vi "Grain Boundary Genie - Copy.vi"() -> ()   [LabVIEW 2010]
uses:
  <vilib>/Analysis/NI_AALBase.lvlib
  <vilib>/Analysis/baseanly.llb/Real Dot Product.vi
  <vilib>/Analysis/NI_AALPro.lvlib
  <vilib>/Analysis/_algsub.llb/Real Vector Norm.vi
  <vilib>/picture/3D Picture Control/NI_3D Picture Control.lvlib
  <vilib>/Analysis/baseanly.llb/Real A x B.vi
  <vilib>/Analysis/baseanly.llb/Vector x A.vi
  <vilib>/Utility/file.llb/Write To Spreadsheet File (string).vi
panel:
  in  "Grain 2 Max Length (A)":dbl=10.0
  in  "Grain 1 Max Length (A)":dbl=10.0
  in  "Max Grain Width":dbl=100.0
  in  "Grain 1 Start":dbl
  in  "Conventional Unit Cell":T1={"Structure Name"="CdTe", "Lattice vector a"=[6.615785553057252, 0.0, 0.0], "Lattice vector b"=[0.0, 6.615785553057252, 0.0], "Lattice vector c"=[0.0, 0.0, 6.615785553057252], "Atoms Array"=[{"Atom Name"="Cd", "Positions (Direct)"=[[0.0, 0.0, 0.0], [0.0, 0.5, 0.5], [0.5, 0.0, 0.5], [0.5, 0.5, 0.0]], "Positions (Cartesian)"=[[0.0, 0.0, 0.0], [0.0, 3.307892776528626, 3.307892776528626], [3.307892776528626, 0.0, 3.307892776528626], [3.307892776528626, 3.307892776528626, 0.0]]}, {"Atom Name"="Te", "Positions (Direct)"=[[0.25, 0.25, 0.25], [0.75, 0.75, 0.25], [0.75, 0.25, 0.75], [0.25, 0.75, 0.75]], "Positions (Cartesian)"=[[1.653946388264313, 1.653946388264313, 1.653946388264313], [4.96183916479294, 4.96183916479294, 1.653946388264313], [4.96183916479294, 1.653946388264313, 4.96183916479294], [1.653946388264313, 4.96183916479294, 4.96183916479294]]}], "# of atoms"=8}
  in  "Overlap Region (A)":dbl(slide) scale=-2.0..1.0
  in  "Tab Control":T2(tab)
  in  "Remove Close Atoms":bool
  out "Subset for Y?":bool
  out "Repeating Y Length Scale":dbl=99.01964045547014
  in  "Crop to Smallest Repeating":bool
  in  "Slab Y":dbl=6.0
  in  "Slab X":dbl=6.0
  out "Subset for X?":bool
  in  "Tolerance (A)":dbl=1.0
  in  "Presorted?":bool
  out "Repeating X Length Scale":dbl=99.01964045547014
  in  "Minimally Allowable Distance (A)":dbl=1.5
  out "# of Atoms Removed":i32
  in  "Make GB":bool
  in  "Options":cluster{"Border?":bool, "Bonds?":bool}={"Border?"=TRUE, "Bonds?"=FALSE}
  in  "Scale":dbl(slide)=0.06161137440758294 scale=0.0..0.2
  in  "Mutual Viewing Angle":dbl[](array[numeric])=[1.0, 0.0, 0.0]
  out "# of Atoms":i32
  out "Atoms / A³":dbl
  out "% of Bulk atomic density":dbl
  in  "Structure Name":string
  in  "Save to POSCAR":bool
  out "Grain Boundary Object":refnum<vi>
  out "Grain 2 Object":refnum<vi>
  out "Grain 1 Object":refnum<vi>
  in  "Add Tilt Angle":dbl(slide) scale=0.0..90.0
  out "Grain Boundary":T1={"Structure Name"="Relax2 Subcrystal Expanded to Box+Relax2 Subcrystal Expanded to Box", "Lattice vector a"=[10.1, 0.0, 0.0], "Lattice vector b"=[0.0, 100.1, 0.0], "Lattice vector c"=[0.0, 0.0, 24.72380952380952], "Atoms Array"=[{"Atom Name"="Cd", "Positions (Direct)"=array496x3[1488 elements], "Positions (Cartesian)"=array496x3[1488 elements]}, {"Atom Name"="Te", "Positions (Direct)"=array480x3[1440 elements], "Positions (Cartesian)"=array480x3[1440 elements]}], "# of atoms"=976} {"Atoms Array"."Positions (Cartesian)" format="%#_4f"; "Atoms Array"."Positions (Direct)" format="%#_4f"}
  out "Grain 2":T1={"Structure Name"="Relax2 Subcrystal Expanded to Box", "Lattice vector a"=[10.1, 0.0, 0.0], "Lattice vector b"=[0.0, 100.1, 0.0], "Lattice vector c"=[0.0, 0.0, 10.1], "Atoms Array"=[{"Atom Name"="Cd", "Positions (Direct)"=array248x3[744 elements], "Positions (Cartesian)"=array248x3[744 elements]}, {"Atom Name"="Te", "Positions (Direct)"=array240x3[720 elements], "Positions (Cartesian)"=array240x3[720 elements]}], "# of atoms"=488} {"Atoms Array"."Positions (Cartesian)" format="%#_4f"; "Atoms Array"."Positions (Direct)" format="%#_4f"}
  out "Grain 1":T1={"Structure Name"="Relax2 Subcrystal Expanded to Box", "Lattice vector a"=[10.1, 0.0, 0.0], "Lattice vector b"=[0.0, 100.1, 0.0], "Lattice vector c"=[0.0, 0.0, 10.1], "Atoms Array"=[{"Atom Name"="Cd", "Positions (Direct)"=array248x3[744 elements], "Positions (Cartesian)"=array248x3[744 elements]}, {"Atom Name"="Te", "Positions (Direct)"=array240x3[720 elements], "Positions (Cartesian)"=array240x3[720 elements]}], "# of atoms"=488} {"Atoms Array"."Positions (Cartesian)" format="%#_4f"; "Atoms Array"."Positions (Direct)" format="%#_4f"}
  in  "Primitive Lattice Vectors":T1={"Structure Name"="Relax2 Subcrystal", "Lattice vector a"=[0.0, 3.3046962263585, 3.3046962263585], "Lattice vector b"=[3.3046962263585, 0.0, 3.3046962263585], "Lattice vector c"=[3.3046962263585, 3.3046962263585, 0.0], "Atoms Array"=[{"Atom Name"="Cd", "Positions (Direct)"=[[0.0, 0.0, 0.0]], "Positions (Cartesian)"=[[0.0, 0.0, 0.0]]}, {"Atom Name"="Te", "Positions (Direct)"=[[0.25, 0.25, 0.25]], "Positions (Cartesian)"=[[1.65234811317925, 1.65234811317925, 1.65234811317925]]}], "# of atoms"=2} {"Atoms Array"."Positions (Cartesian)" format="%#_4f"; "Atoms Array"."Positions (Direct)" format="%#_4f"}
  in  "Grain 2 Min Length (A)":dbl=10.0
  in  "Grain 1 Min Length (A)":dbl=10.0
  out "Grain Boundary Render":refnum<vi>(3d-picture)
  in  "Max Grain Height":dbl=100.0
  in  "Translation Vector":dbl[](array[slide])=[0.0, 0.0, 4.523809523809524] scale=0.0..2.0
  in  "Twist Angle":dbl(slide)=60.0 scale=0.0..60.0
  in  "Grain 2 Orientation":dbl[](array[numeric])=[1.0, 0.0, 0.0]
  in  "Grain 1 Orientation":dbl[](array[numeric])=[1.0, 0.0, 0.0]
  out "Grain 2 Render":refnum<vi>(3d-picture)
  out "Grain 1 Render":refnum<vi>(3d-picture)
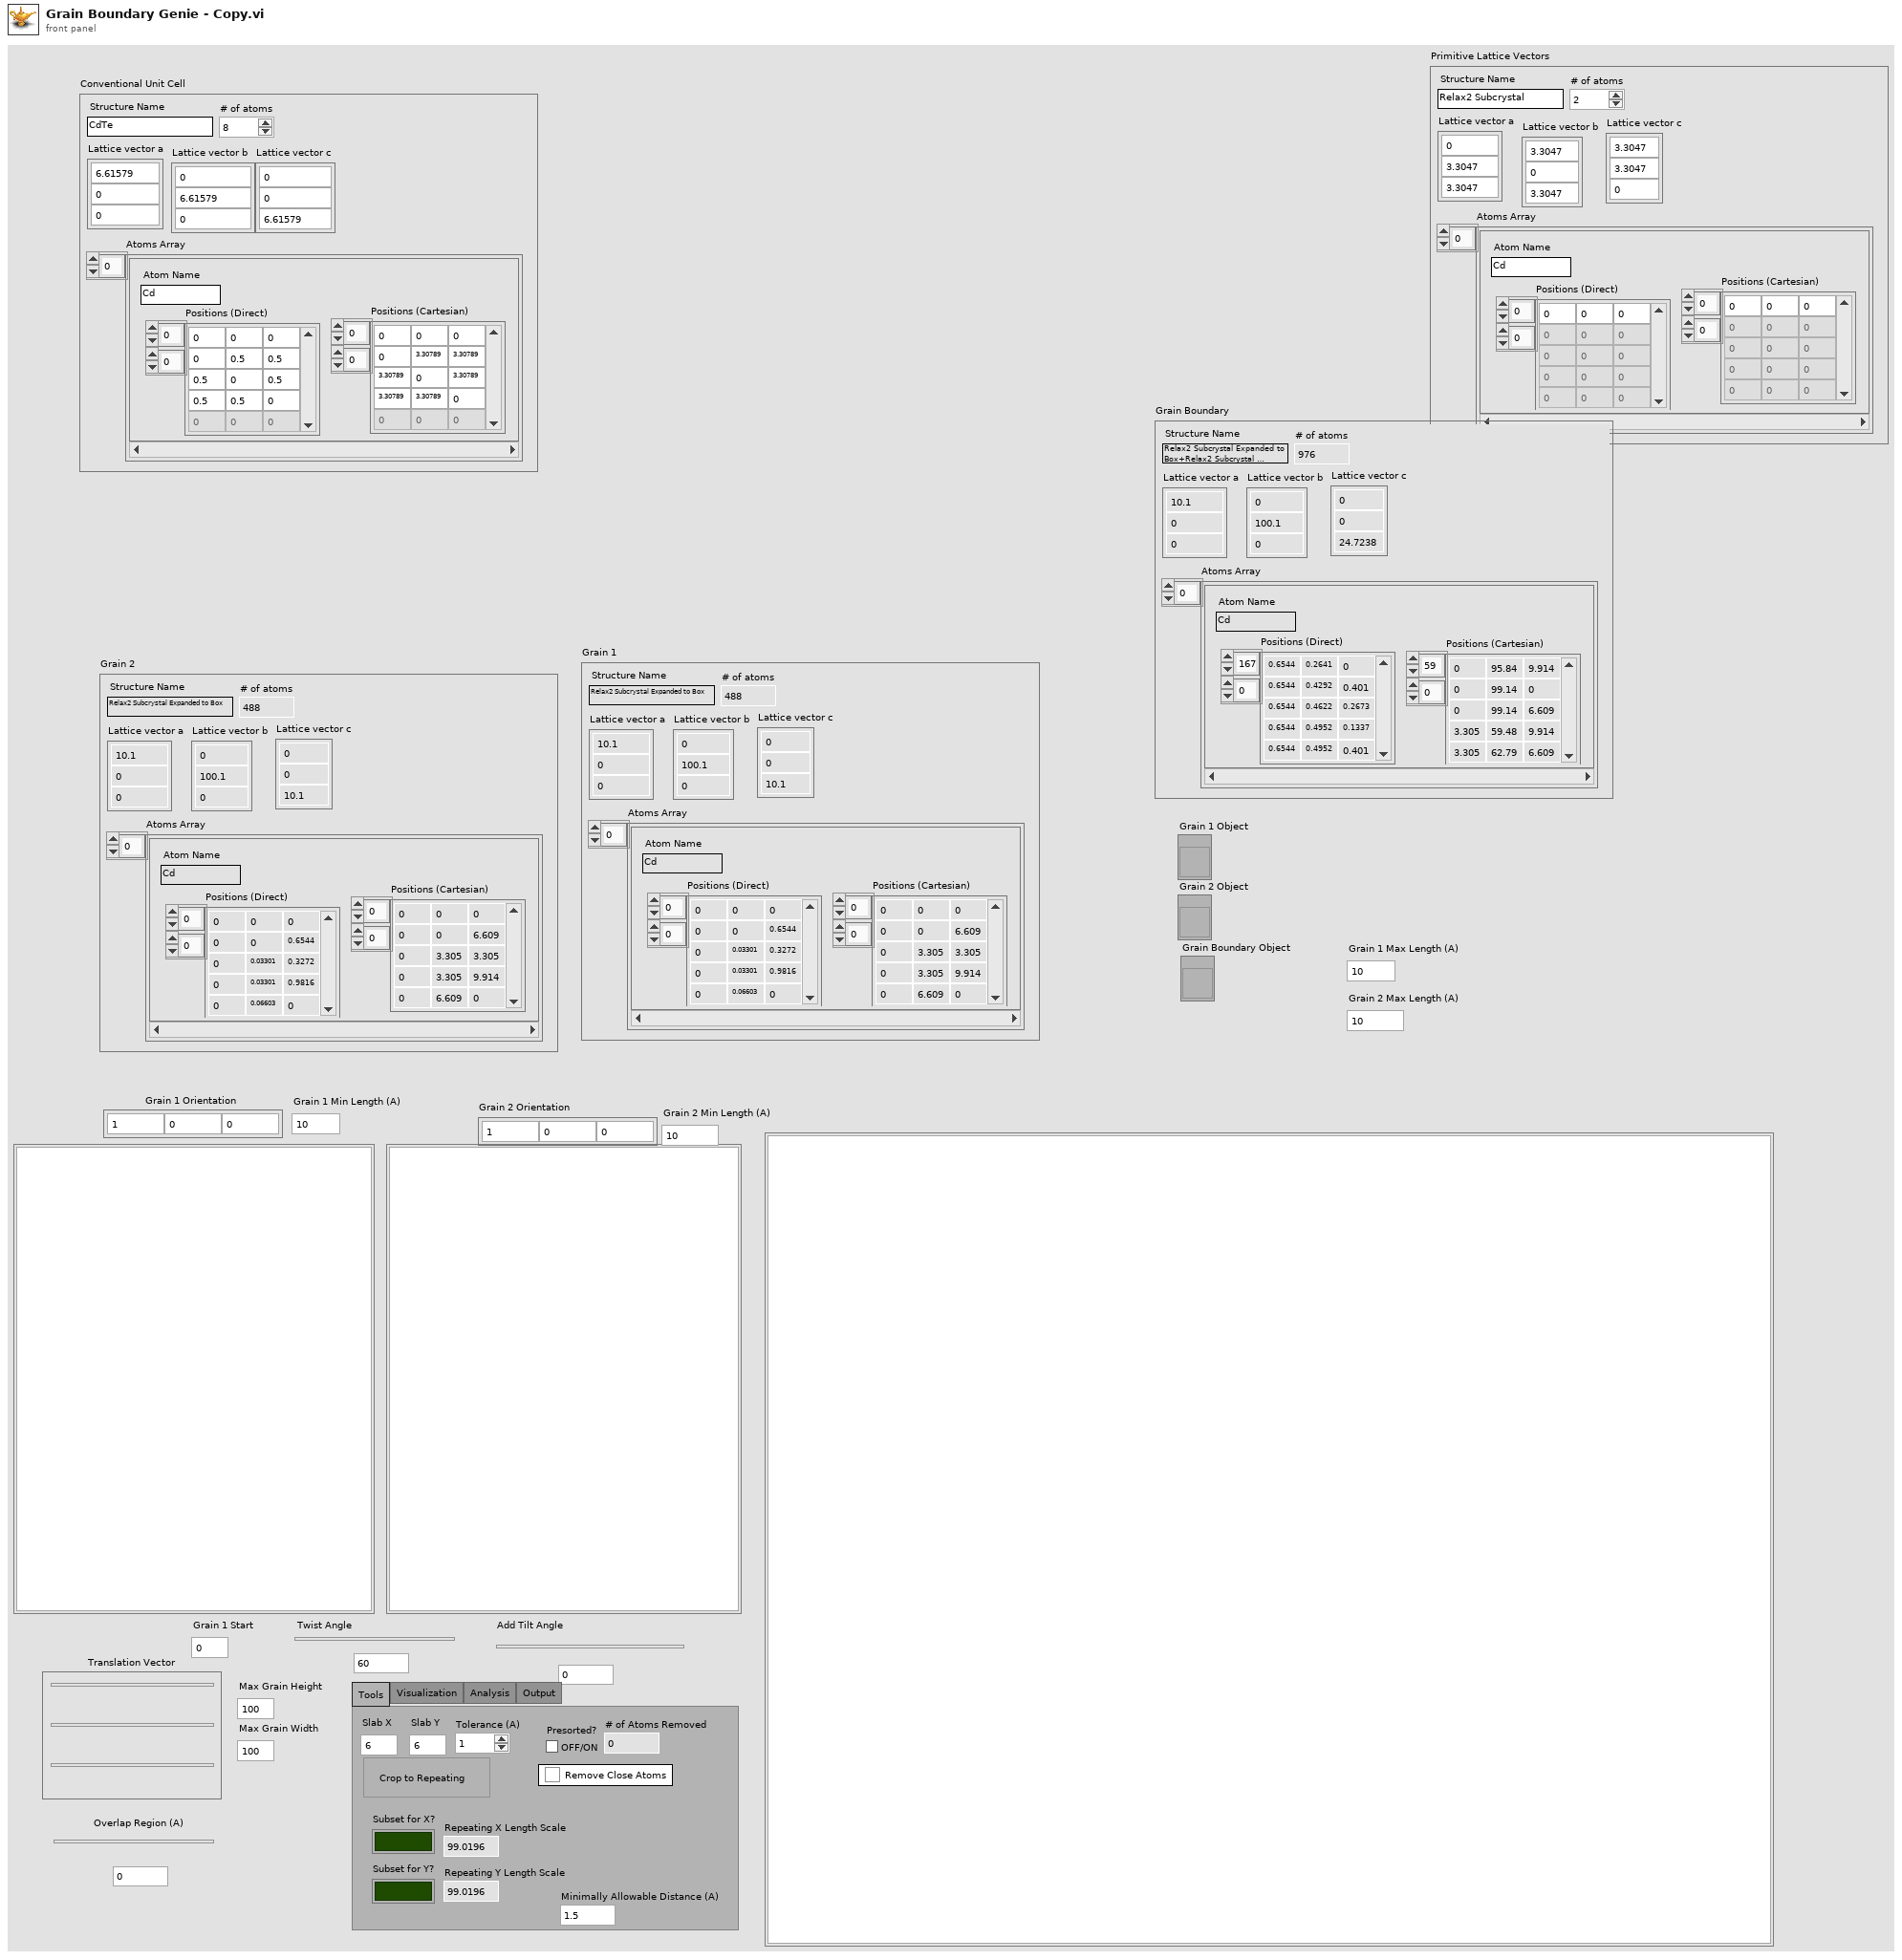
[diagram p1: front panel]
types:
  T1 = cluster{"Structure Name":string, "Lattice vector a":dbl[], "Lattice vector b":dbl[], "Lattice vector c":dbl[], "Atoms Array":cluster{"Atom Name":string, "Positions (Direct)":dbl[][], "Positions (Cartesian)":dbl[][]}[], "# of atoms":i32}
  T2 = enum32{"Tools", "Visualization", "Analysis", "Output"}
  T3 = typedef "NI_Matrix.lvlib/RealMatrix.ctl" = dbl[][]
  T4 = cluster{"Z Min":dbl, "Max Grain Width":dbl, "Z Min":dbl, "Max Grain Height":dbl, "Grain 1 Start":dbl, "Grain 1 Min Length (A)":dbl}
  T5 = cluster{"Grain 1 Start":dbl, "Max Grain Width":dbl, "Grain 1 Start":dbl, "Max Grain Height":dbl, dbl, "Grain 2 Min Length (A)":dbl}
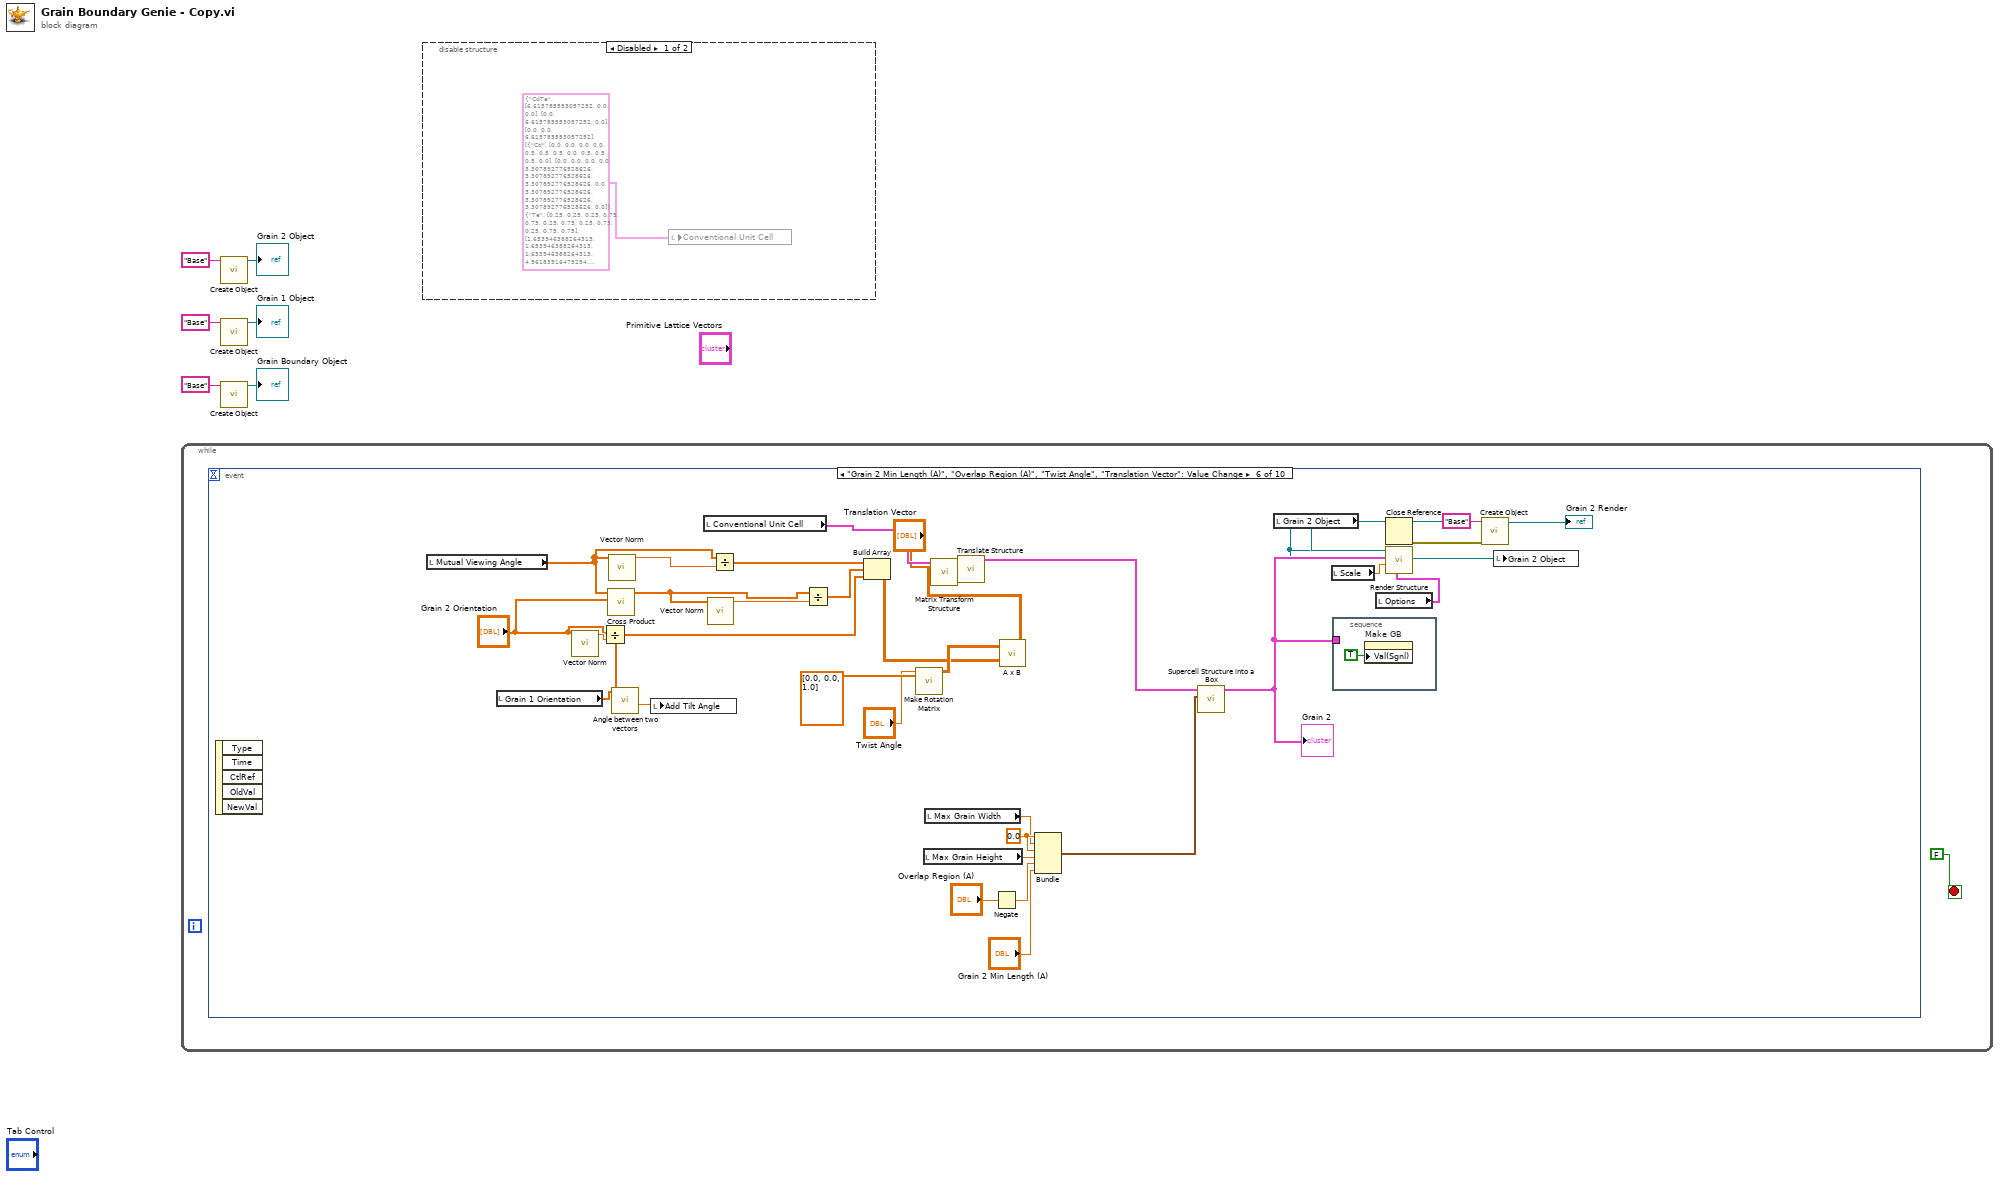
[diagram p0: block diagram]
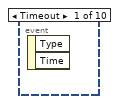
[diagram p3: hidden frame]
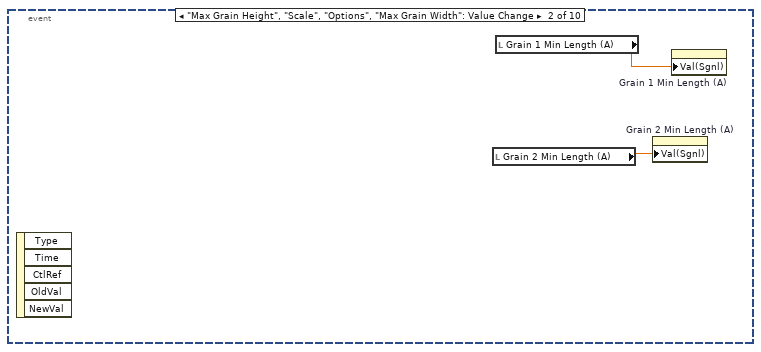
[diagram p4: hidden frame]
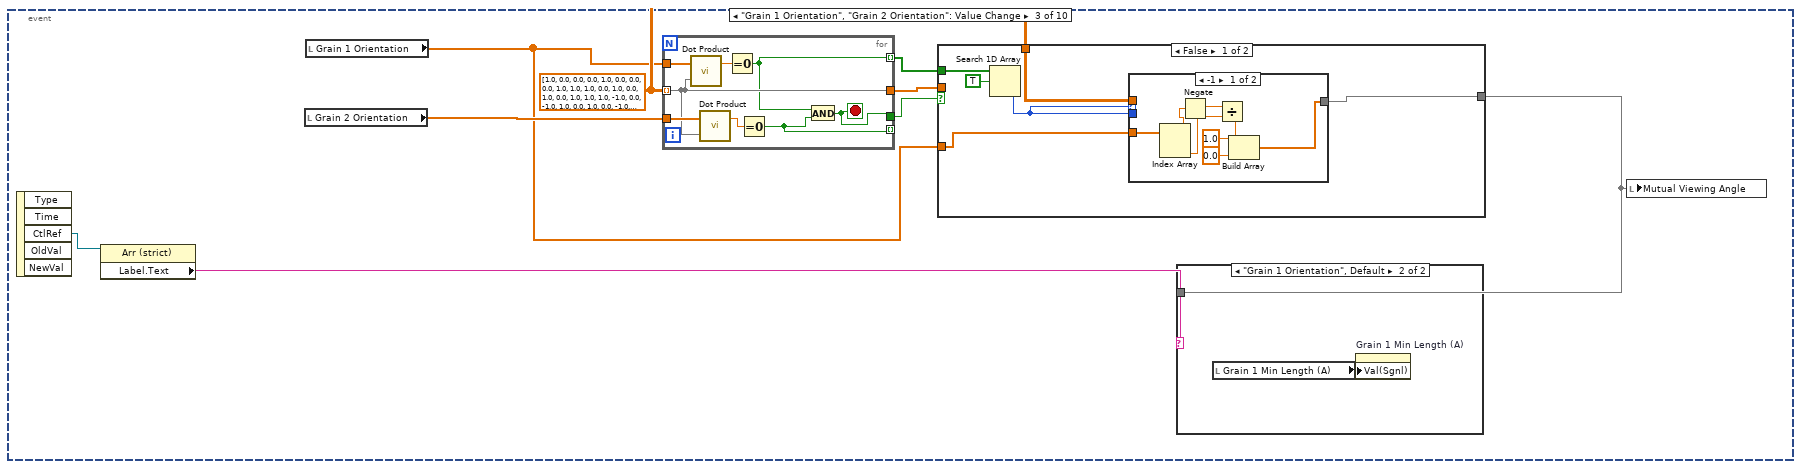
[diagram p5: hidden frame]
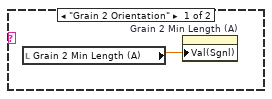
[diagram p6: hidden frame]
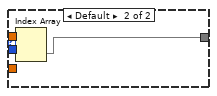
[diagram p7: hidden frame]
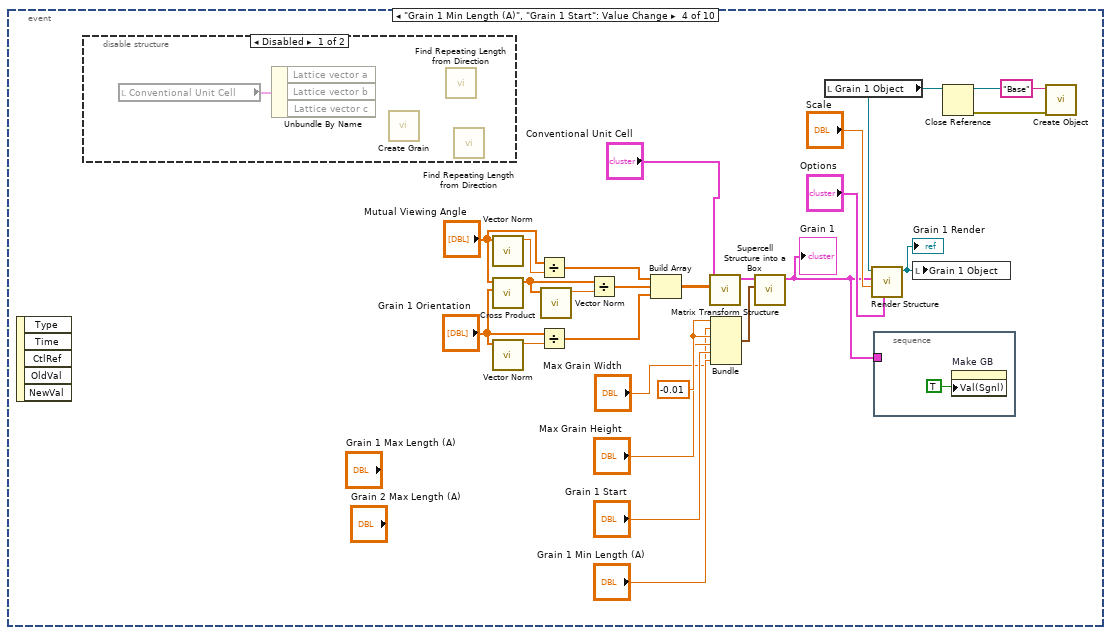
[diagram p9: hidden frame]
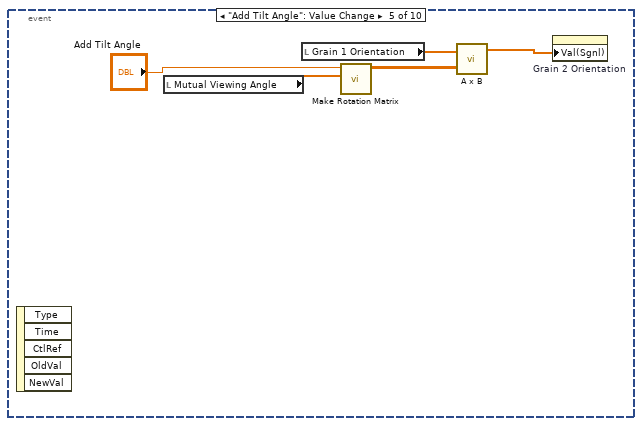
[diagram p11: hidden frame]
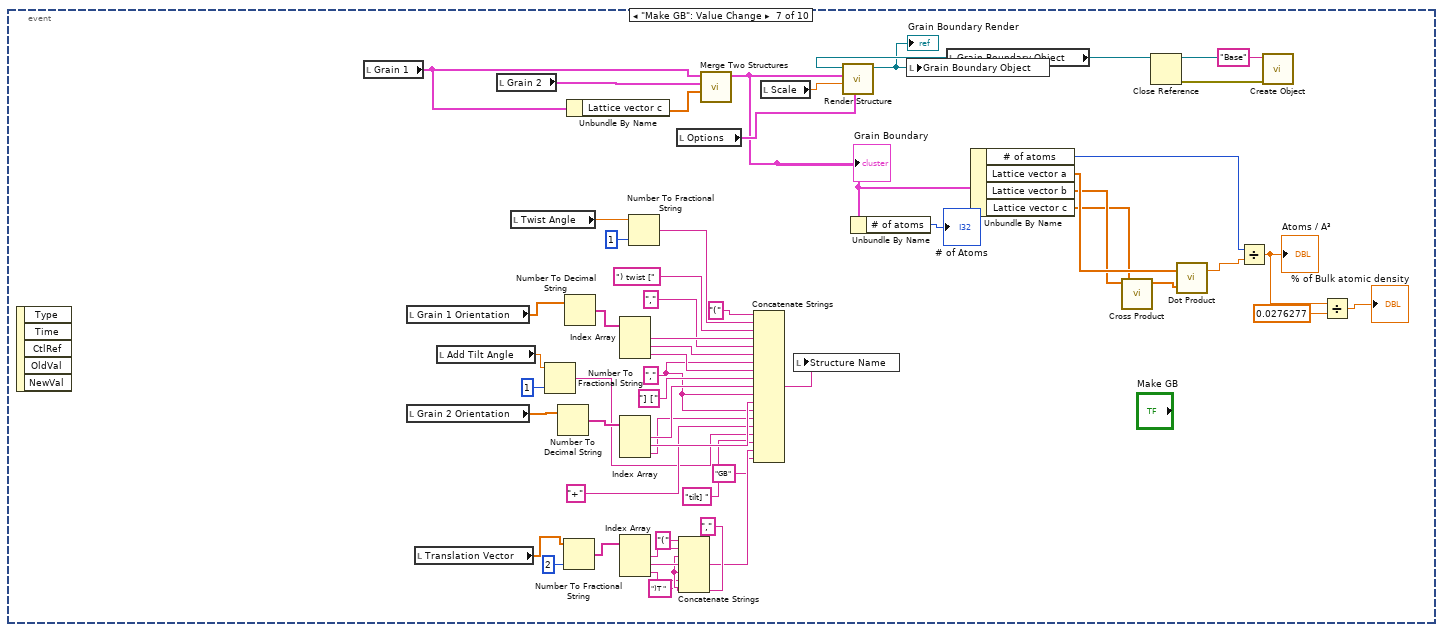
[diagram p12: hidden frame]
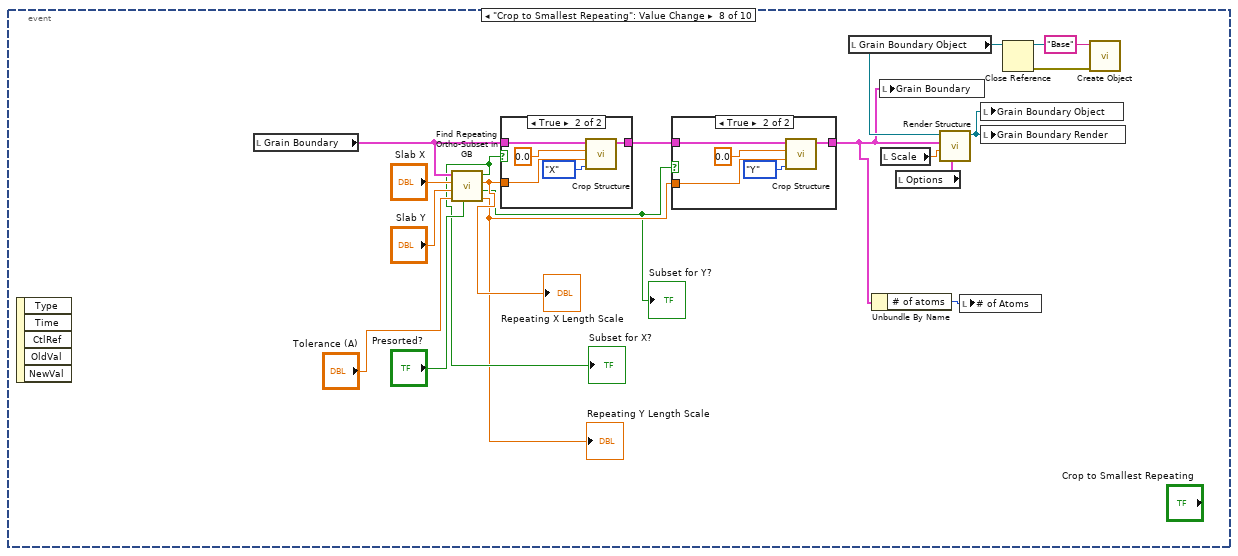
[diagram p13: hidden frame]
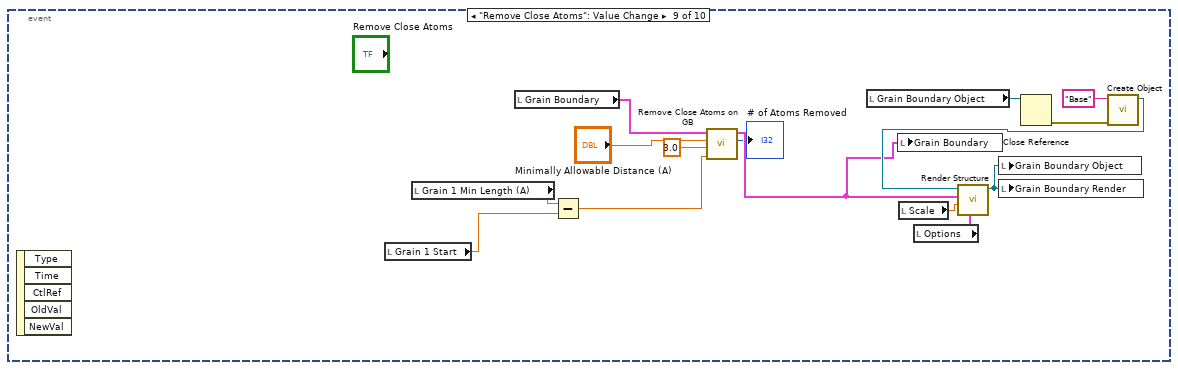
[diagram p16: hidden frame]
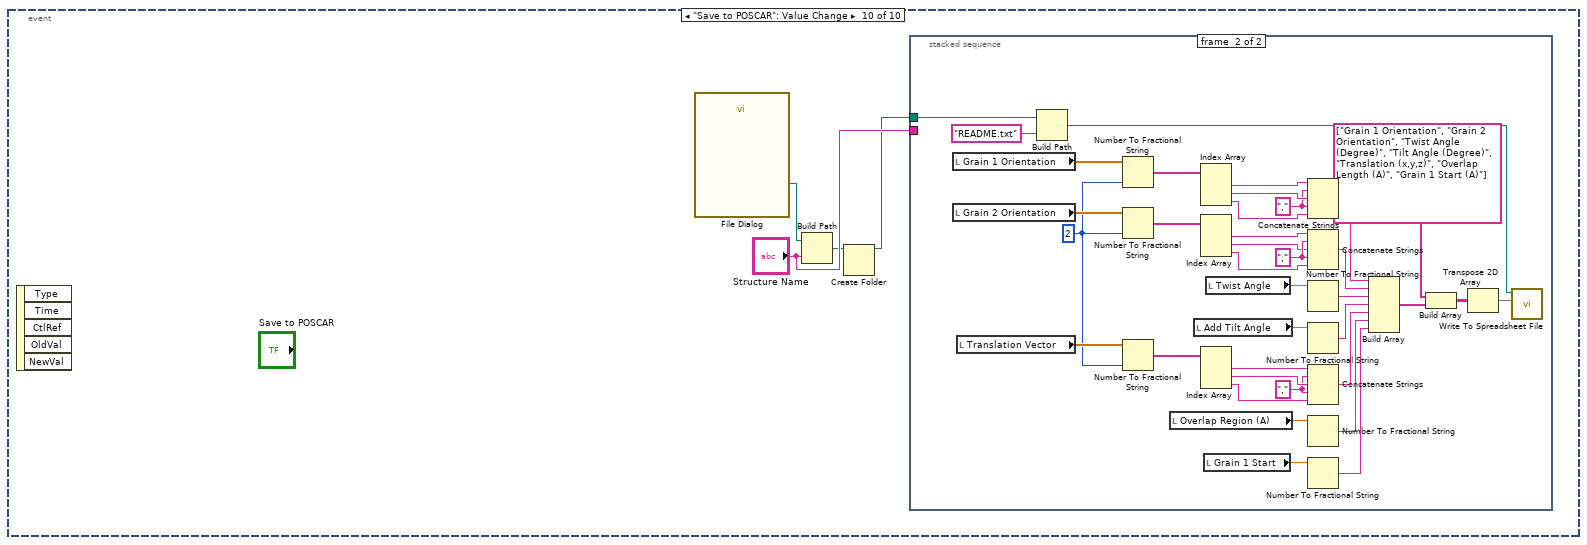
[diagram p17: hidden frame]
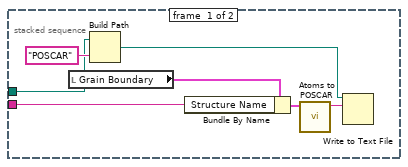
[diagram p18: hidden frame]
diagram:
  n1 = while {
    stop <- FALSE stop-if-true
    n2 = event shown="[5] \"Grain 2 Min Length (A)\", \"Overlap Region (A)\", \"Twist Angle\", \"Translation Vector\": Value Change" {
      selector: _ -> [_ _ _ _ _ _ _ _ _ _]
      dyn-events: _ -> [_ _ _ _ _ _ _ _ _ _]
      timeout: _ -> [_ _ _ _ _ _ _ _ _ _]
      event Timeout {
        n3 = event-data() -> ()  [unwired: 1 in, 2 out]
      }
      event "Max Grain Height", "Scale", "Options", "Max Grain Width": Value Change {
        n4 = event-data() -> ()  [unwired: 1 in, 5 out]
        n5 = local read "Grain 2 Min Length (A)"() -> (w8:dbl)
        n6 = local read "Grain 1 Min Length (A)"() -> (w9:dbl)
        n7 = property on="Grain 2 Min Length (A)" class="DigNum (strict)"("Val(Sgnl)"=w8) -> ()  [unwired: 2 in, 2 out]
        n8 = property on="Grain 1 Min Length (A)" class="DigNum (strict)"("Val(Sgnl)"=w9) -> ()  [unwired: 2 in, 2 out]
      }
      event "Grain 1 Orientation", "Grain 2 Orientation": Value Change {
        w14 = dbl[][] [[1.0, 0.0, 0.0], [0.0, 1.0, 0.0], [0.0, 0.0, 1.0], [1.0, 1.0, 0.0], [1.0, 0.0, 1.0], [0.0, 1.0, 1.0], [1.0, -1.0, 0.0], [-1.0, 1.0, 0.0], [1.0, 0.0, -1.0], [-1.0, 0.0, 1.0], [0.0, -1.0, 1.0], [0.0, 1.0, -1.0], [2.0, 1.0, 0.0], [2.0, 1.0, 1.0]] ("Grain 1 Orientation 2")
        n9 = event-data() -> ("CtlRef"=w13:refnum<vi>)  [unwired: 1 in, 4 out]
        n10 = property class="Arr (strict)"(reference=w13) -> ("Label.Text"=w12:string)  [unwired: 1 in, 2 out]
        n11 = local read "Grain 2 Orientation"() -> (w18:dbl[])
        n12 = local read "Grain 1 Orientation"() -> (w11:dbl[])
        n13 = for {
          tunnel: w11 -> [w46]
          tunnel: w14 -> [w43] mode=indexing
          tunnel: [w43] -> w16
          tunnel: w18 -> [w44]
          tunnel: [w41] -> w15 mode=indexing
          tunnel: [w40] -> _ mode=indexing
          tunnel: [w39] -> w17
          stop <- w39 stop-if-true
          n14 = call-poly <vilib>:"Dot Product.vi"("Y Vector"=w43, "X Vector"=w46) -> ("X * Y"=w45:dbl)  [unwired: 1 out]
          n15 = call-poly <vilib>:"Dot Product.vi"("Y Vector"=w43, "X Vector"=w44) -> ("X * Y"=w42:dbl)  [unwired: 1 out]
          n16 = Equal To 0?(x=w45) -> (x = 0?=w41:bool)
          n17 = Equal To 0?(x=w42) -> (x = 0?=w40:bool)
          n18 = And(x=w41, y=w40) -> (x .and. y?=w39:bool)
        }
        n19 = case shown="False" w17 {
          tunnel: w16 -> [_ w38]
          tunnel: [w23 w38] -> w10
          tunnel: w15 -> [w26 _]
          tunnel: w14 -> [w24 _]
          tunnel: w11 -> [w21 _]
          frame False {
            n20 = Search 1D Array(1D array=w26, element=TRUE) -> (index of element=w22:i32)  [unwired: 1 in]
            n21 = case shown="-1" w22 {
              tunnel: w24 -> [_ w37]
              tunnel: w22 -> [_ w36]
              tunnel: [w31 w35] -> w23
              tunnel: w21 -> [w34 _]
              frame -1 {
                n22 = Index Array(array=w34) -> (element #1=w29:dbl, element #2=w30:dbl)  [unwired: 2 in]
                n23 = Negate(x=w29) -> (-x=w28:dbl)
                n24 = Divide(x=w28, y=w30) -> (x/y=w27:dbl)
                n25 = Build Array(1.0 ("element"), w27, 0.0 ("element")) -> (w31:dbl[])
              }
              frame Default {
                n26 = Index Array(array=w37, index (row)=w36) -> (element=w35:dbl[])  [unwired: 1 in]
              }
            }
          }
          frame True {
          }
        }
        n27 = case shown="\"Grain 1 Orientation\", Default" w12 {
          tunnel: w10 -> [_ _]
          frame "Grain 2 Orientation" {
            n28 = local read "Grain 2 Min Length (A)"() -> (w19:dbl)
            n29 = property on="Grain 2 Min Length (A)" class="DigNum (strict)"("Val(Sgnl)"=w19) -> ()  [unwired: 2 in, 2 out]
          }
          frame "Grain 1 Orientation", Default {
            n30 = local read "Grain 1 Min Length (A)"() -> (w20:dbl)
            n31 = property on="Grain 1 Min Length (A)" class="DigNum (strict)"("Val(Sgnl)"=w20) -> ()  [unwired: 2 in, 2 out]
          }
        }
        n32 = local write "Mutual Viewing Angle"(w10) -> ()
      }
      event "Grain 1 Min Length (A)", "Grain 1 Start": Value Change {
        w65 = -0.01 ("Z Min")
        n33 = event-data() -> ()  [unwired: 1 in, 5 out]
        n34 = disable-structure shown="Disabled" {
          frame Disabled {
            n35 = local read "Conventional Unit Cell"() -> (w73:T1)
            n36 = Unbundle By Name(w73) -> ()  [unwired: 3 out]
            n37 = call "Create Grain.vi"() -> ()  [unwired: 11 in, 1 out]
            n38 = call "Find Repeating Length from Direction.vi"() -> ()  [unwired: 11 in, 1 out]
            n39 = call "Find Repeating Length from Direction.vi"() -> ()  [unwired: 11 in, 1 out]
          }
          frame Enabled {
          }
        }
        n40 = call-poly <vilib>:"Vector Norm.vi"("Input Vector"="Mutual Viewing Angle") -> ("norm"=w72:dbl)  [unwired: 9 in, 1 out]
        n41 = call <vilib>:"Cross Product.vi"("B Vector"="Grain 1 Orientation", "A Vector"="Mutual Viewing Angle") -> ("Cross Product"=w50:dbl[])  [unwired: 8 in, 1 out]
        n42 = call-poly <vilib>:"Vector Norm.vi"("Input Vector"="Grain 1 Orientation") -> ("norm"=w70:dbl)  [unwired: 9 in, 1 out]
        n43 = Divide(x="Mutual Viewing Angle", y=w72) -> (x/y=w69:dbl[])
        n44 = Divide(x="Grain 1 Orientation", y=w70) -> (x/y=w68:dbl[])
        n45 = call-poly <vilib>:"Vector Norm.vi"("Input Vector"=w50) -> ("norm"=w71:dbl)  [unwired: 9 in, 1 out]
        n46 = Divide(x=w50, y=w71) -> (x/y=w47:dbl[])
        n47 = Build Array(w69, w47, w68) -> (w67:T3)
        n48 = call "Matrix Transform Structure.vi"("Matrix Transform"=w67, "Original Structure"="Conventional Unit Cell") -> ("After Transform"=w64:T1)  [unwired: 9 in]
        n49 = Bundle("Z Min"=w65, "Max Grain Width"="Max Grain Width", "Z Min"=w65, "Max Grain Height"="Max Grain Height", "Grain 1 Start"="Grain 1 Start", "Grain 1 Min Length (A)"="Grain 1 Min Length (A)") -> (w66:T4)  [unwired: 1 in]
        n50 = call "Supercell Structure into a Box.vi"("Draw Box"=w66, "Subcrystal"=w64) -> ("Expanded cubic Structure"=w56:T1)  [unwired: 7 in, 2 out]
        "Grain 1" <- w56
        n51 = local read "Grain 1 Object"() -> (w55:refnum<vi>)
        n52 = stacked-sequence {
          tunnel: w56 -> [_]
          frame #0 {
            n53 = property on="Make GB" class="Bool (strict)"("Val(Sgnl)"=TRUE ("Value (Signaling)")) -> ()  [unwired: 2 in, 2 out]
          }
        }
        n54 = Close Reference(reference=w55) -> (error out=w54:errorcluster)  [unwired: 1 in]
        n55 = call <vilib>:"Create Object.vi"("error in (no error)"=w54, "Name"="Base") -> ("Scene:New Object"=w60:refnum<vi>)  [unwired: 9 out]
        n56 = call "Render Structure.vi"("Options"="Options", "Scale"="Scale", "Atomic Structure"=w56, "Base Object"=w60) -> ("Object with atoms"=w53:refnum<vi>)  [unwired: 7 in]
        "Grain 1 Render" <- w53
        n57 = local write "Grain 1 Object"(w53) -> ()
      }
      event "Add Tilt Angle": Value Change {
        n58 = event-data() -> ()  [unwired: 1 in, 5 out]
        n59 = local read "Mutual Viewing Angle"() -> (w75:dbl[])
        n60 = local read "Grain 1 Orientation"() -> (w77:dbl[])
        n61 = call "Make Rotation Matrix.vi"("Rotation Axis"=w75, "Rotation Angle (Degree)"="Add Tilt Angle") -> ("Rotation Matrix"=w78:T3)  [unwired: 9 in]
        n62 = call-poly <vilib>:"A x B.vi"("Matrix A"=w78, "Vector V'"=w77) -> ("V' x A"=w76:dbl[])  [unwired: 1 out]
        n63 = property on="Grain 2 Orientation" class="Arr (strict)"("Val(Sgnl)"=w76) -> ()  [unwired: 2 in, 2 out]
      }
      event "Grain 2 Min Length (A)", "Overlap Region (A)", "Twist Angle", "Translation Vector": Value Change {
        w107 = 0.0 ("Grain 1 Start")
        n64 = event-data() -> ()  [unwired: 1 in, 5 out]
        n65 = local read "Mutual Viewing Angle"() -> (w81:dbl[])
        n66 = local read "Grain 1 Orientation"() -> (w87:dbl[])
        n67 = call-poly <vilib>:"Vector Norm.vi"("Input Vector"="Grain 2 Orientation") -> ("norm"=w112:dbl)  [unwired: 9 in, 1 out]
        n68 = Divide(x="Grain 2 Orientation", y=w112) -> (x/y=w110:dbl[])
        n69 = call <vilib>:"Cross Product.vi"("B Vector"="Grain 2 Orientation", "A Vector"=w81) -> ("Cross Product"=w109:dbl[])  [unwired: 8 in, 1 out]
        n70 = call-poly <vilib>:"Vector Norm.vi"("Input Vector"=w81) -> ("norm"=w114:dbl)  [unwired: 9 in, 1 out]
        n71 = call "Angle between two vectors.vi"("Vector 2"="Grain 2 Orientation", "Vector 1"=w87) -> ("Angle (Degrees)"=w86:dbl)  [unwired: 7 in, 2 out]
        n72 = local write "Add Tilt Angle"(w86) -> ()
        n73 = local read "Conventional Unit Cell"() -> (w85:T1)
        n74 = call-poly <vilib>:"Vector Norm.vi"("Input Vector"=w109) -> ("norm"=w113:dbl)  [unwired: 9 in, 1 out]
        n75 = Divide(x=w81, y=w114) -> (x/y=w111:dbl[])
        n76 = Divide(x=w109, y=w113) -> (x/y=w80:dbl[])
        n77 = Build Array(w111, w80, w110) -> (w90:T3)
        n78 = call "Make Rotation Matrix.vi"("Rotation Axis"=dbl[] [0.0, 0.0, 1.0], "Rotation Angle (Degree)"="Twist Angle") -> ("Rotation Matrix"=w91:T3)  [unwired: 9 in]
        n79 = local read "Max Grain Height"() -> (w104:dbl)
        n80 = local read "Max Grain Width"() -> (w89:dbl)
        n81 = Negate(x="Overlap Region (A)") -> (-x=w95:dbl)
        n82 = call-poly <vilib>:"A x B.vi"("B"=w90, "A"=w91) -> ("A x B"=w92:T3)  [unwired: 1 out]
        n83 = call "Matrix Transform Structure.vi"("Matrix Transform"=w92, "Original Structure"=w85) -> ("After Transform"=w84:T1)  [unwired: 9 in]
        n84 = call "Translate Structure.vi"("Translation Vector (Cartesian)"="Translation Vector", "Atomic Structure"=w84) -> ("Shifted Structure"=w82:T1)  [unwired: 9 in]
        n85 = Bundle("Grain 1 Start"=w107, "Max Grain Width"=w89, "Grain 1 Start"=w107, "Max Grain Height"=w104, w95, "Grain 2 Min Length (A)"="Grain 2 Min Length (A)") -> (w108:T5)  [unwired: 1 in]
        n86 = call "Supercell Structure into a Box.vi"("Draw Box"=w108, "Subcrystal"=w82) -> ("Expanded cubic Structure"=w100:T1)  [unwired: 7 in, 2 out]
        "Grain 2" <- w100
        n87 = local read "Grain 2 Object"() -> (w98:refnum<vi>)
        n88 = local read "Scale"() -> (w102:dbl)
        n89 = stacked-sequence {
          tunnel: w100 -> [_]
          frame #0 {
            n90 = property on="Make GB" class="Bool (strict)"("Val(Sgnl)"=TRUE ("Value (Signaling)")) -> ()  [unwired: 2 in, 2 out]
          }
        }
        n91 = local read "Options"() -> (w101:cluster{"Border?":bool, "Bonds?":bool})
        n92 = Close Reference(reference=w98) -> (error out=w97:errorcluster)  [unwired: 1 in]
        n93 = call <vilib>:"Create Object.vi"("error in (no error)"=w97, "Name"="Base") -> ("Scene:New Object"=w105:refnum<vi>)  [unwired: 9 out]
        n94 = call "Render Structure.vi"("Options"=w101, "Scale"=w102, "Atomic Structure"=w100, "Base Object"=w105) -> ("Object with atoms"=w99:refnum<vi>)  [unwired: 7 in]
        "Grain 2 Render" <- w99
        n95 = local write "Grain 2 Object"(w99) -> ()
      }
      event "Make GB": Value Change {
        w130 = "," ("string")
        w149 = "," ("string")
        n96 = event-data() -> ()  [unwired: 1 in, 5 out]
        n97 = local read "Grain 1"() -> (w166:T1)
        n98 = local read "Grain 1 Orientation"() -> (w147:dbl[])
        n99 = local read "Grain 2 Orientation"() -> (w145:dbl[])
        n100 = local read "Translation Vector"() -> (w136:dbl[])
        n101 = local read "Add Tilt Angle"() -> (w143:dbl)
        n102 = local read "Grain 2"() -> (w171:T1)
        n103 = local read "Twist Angle"() -> (w161:dbl)
        n104 = Number To Fractional String(number=w143, precision (6)=i16 1) -> (F-format string=w141:string)  [unwired: 2 in]
        n105 = Number To Decimal String(number=w145) -> (decimal integer string=w144:string[])  [unwired: 1 in]
        n106 = Number To Fractional String(number=w136, precision (6)=i16 2) -> (F-format string=w134:string[])  [unwired: 2 in]
        n107 = Number To Decimal String(number=w147) -> (decimal integer string=w146:string[])  [unwired: 1 in]
        n108 = Unbundle By Name(w166) -> ("Lattice vector c"=w138:dbl[])
        n109 = Index Array(array=w146) -> (element #1=w157:string, element #2=w155:string, element #3=w154:string)  [unwired: 3 in]
        n110 = Index Array(array=w144) -> (element #1=w152:string, element #2=w150:string, element #3=w148:string)  [unwired: 3 in]
        n111 = Index Array(array=w134) -> (element #1=w133:string, element #2=w131:string, element #3=w129:string)  [unwired: 3 in]
        n112 = Number To Fractional String(number=w161, precision (6)=i16 1) -> (F-format string=w159:string)  [unwired: 2 in]
        n113 = local read "Options"() -> (w167:cluster{"Border?":bool, "Bonds?":bool})
        n114 = Concatenate Strings("(" ("string"), w133, w130, w131, w130, w129, ")T " ("string")) -> (w127:string)
        n115 = call "Merge Two Structures.vi"("Translation Vector (1 to 2)"=w138, "Atomic Structure 2"=w171, "Atomic Structure 1"=w166) -> ("Atomic Structure of 1 + 2 by T"=w125:T1)  [unwired: 8 in]
        "Grain Boundary" <- w125
        n116 = Concatenate Strings("(" ("string"), w159, ") twist [" ("string"), w157, "," ("string"), w155, w149, w154, "] [" ("string"), w152, w149, w150, w149, w148, "+" ("string"), w141, "tilt] " ("string"), w127, "GB" ("string")) -> (w151:string)
        n117 = local read "Scale"() -> (w168:dbl)
        n118 = local write "Structure Name"(w151) -> ()
        n119 = Unbundle By Name(w125) -> ("# of atoms"=→"# of Atoms":i32)
        n120 = local read "Grain Boundary Object"() -> (w164:refnum<vi>)
        n121 = Unbundle By Name(w125) -> ("# of atoms"=w119:i32, "Lattice vector a"=w124:dbl[], "Lattice vector b"=w123:dbl[], "Lattice vector c"=w122:dbl[])
        n122 = call <vilib>:"Cross Product.vi"("B Vector"=w122, "A Vector"=w123) -> ("Cross Product"=w121:dbl[])  [unwired: 8 in, 1 out]
        n123 = Close Reference(reference=w164) -> (error out=w163:errorcluster)  [unwired: 1 in]
        n124 = call-poly <vilib>:"Dot Product.vi"("Y Vector"=w121, "X Vector"=w124) -> ("X * Y"=w120:dbl)  [unwired: 1 out]
        n125 = Divide(x=w119, y=w120) -> (x/y=w118:dbl)
        "Atoms / A³" <- w118
        n126 = call <vilib>:"Create Object.vi"("error in (no error)"=w163, "Name"="Base") -> ("Scene:New Object"=w169:refnum<vi>)  [unwired: 9 out]
        n127 = call "Render Structure.vi"("Options"=w167, "Scale"=w168, "Atomic Structure"=w125, "Base Object"=w169) -> ("Object with atoms"=w165:refnum<vi>)  [unwired: 7 in]
        "Grain Boundary Render" <- w165
        n128 = local write "Grain Boundary Object"(w165) -> ()
        n129 = Divide(x=w118, y=0.0276277) -> (x/y=→"% of Bulk atomic density":dbl)
      }
      event "Crop to Smallest Repeating": Value Change {
        n130 = event-data() -> ()  [unwired: 1 in, 5 out]
        n131 = local read "Grain Boundary"() -> (w183:T1)
        n132 = call "Find Repeating Ortho-Subset in GB.vi"("Presorted?"="Presorted?", "Tolerance (A)"="Tolerance (A)", "Slab Y"="Slab Y", "Slab X"="Slab X", "Grain Boundary"=w183) -> ("Repeating Y Length Scale"=w175:dbl, "Subset Y found?!"=w174:bool, "Repeating X Length Scale"=w177:dbl, "Subset X found?!"=w176:bool)  [unwired: 3 in]
        "Repeating X Length Scale" <- w177
        "Subset for X?" <- w176
        "Repeating Y Length Scale" <- w175
        "Subset for Y?" <- w174
        n133 = case shown="True" w176 {
          tunnel: w183 -> [w197 w202]
          tunnel: [w197 w199] -> w178
          tunnel: w177 -> [_ w198]
          frame False {
          }
          frame True {
            n134 = call "Crop Structure.vi"("Cropping Index"=enum16{"X", "Y", "Z"}."X", "Upper Bound Z"=w198, "Lower bound Z"=0.0, "Input Structure"=w202) -> ("Cropped Structure"=w199:T1)  [unwired: 7 in]
          }
        }
        n135 = case shown="True" w174 {
          tunnel: w178 -> [w191 w196]
          tunnel: w175 -> [_ w194]
          tunnel: [w191 w192] -> w173
          frame False {
          }
          frame True {
            n136 = call "Crop Structure.vi"("Cropping Index"=enum16{"X", "Y", "Z"}."Y", "Upper Bound Z"=w194, "Lower bound Z"=0.0, "Input Structure"=w196) -> ("Cropped Structure"=w192:T1)  [unwired: 7 in]
          }
        }
        n137 = local read "Grain Boundary Object"() -> (w186:refnum<vi>)
        n138 = Unbundle By Name(w173) -> ("# of atoms"=w172:i32)
        n139 = local write "Grain Boundary"(w173) -> ()
        n140 = local read "Scale"() -> (w187:dbl)
        n141 = local read "Options"() -> (w188:cluster{"Border?":bool, "Bonds?":bool})
        n142 = local write "# of Atoms"(w172) -> ()
        n143 = Close Reference(reference=w186) -> (error out=w184:errorcluster)  [unwired: 1 in]
        n144 = call <vilib>:"Create Object.vi"("error in (no error)"=w184, "Name"="Base") -> ("Scene:New Object"=w189:refnum<vi>)  [unwired: 9 out]
        n145 = call "Render Structure.vi"("Options"=w188, "Scale"=w187, "Atomic Structure"=w173, "Base Object"=w189) -> ("Object with atoms"=w185:refnum<vi>)  [unwired: 7 in]
        n146 = local write "Grain Boundary Object"(w185) -> ()
        n147 = local write "Grain Boundary Render"(w185) -> ()
      }
      event "Remove Close Atoms": Value Change {
        n148 = event-data() -> ()  [unwired: 1 in, 5 out]
        n149 = local read "Grain 1 Start"() -> (w205:dbl)
        n150 = local read "Grain 1 Min Length (A)"() -> (w206:dbl)
        n151 = local read "Grain Boundary"() -> (w211:T1)
        n152 = Subtract(x=w206, y=w205) -> (x-y=w204:dbl)
        n153 = call "Remove Close Atoms on GB.vi"("Grain Boundary Location (A)"=w204, "Edge Duplication Range"=3.0, "Minimally Allowable Distance (A)"="Minimally Allowable Distance (A)", "Structure"=w211) -> ("# of Atoms Removed"=→"# of Atoms Removed":i32, "Structure with atoms removed"=w209:T1)  [unwired: 6 in]
        n154 = local read "Grain Boundary Object"() -> (w214:refnum<vi>)
        n155 = local write "Grain Boundary"(w209) -> ()
        n156 = local read "Scale"() -> (w215:dbl)
        n157 = local read "Options"() -> (w216:cluster{"Border?":bool, "Bonds?":bool})
        n158 = Close Reference(reference=w214) -> (error out=w212:errorcluster)  [unwired: 1 in]
        n159 = call <vilib>:"Create Object.vi"("error in (no error)"=w212, "Name"="Base") -> ("Scene:New Object"=w210:refnum<vi>)  [unwired: 9 out]
        n160 = call "Render Structure.vi"("Options"=w216, "Scale"=w215, "Atomic Structure"=w209, "Base Object"=w210) -> ("Object with atoms"=w213:refnum<vi>)  [unwired: 7 in]
        n161 = local write "Grain Boundary Object"(w213) -> ()
        n162 = local write "Grain Boundary Render"(w213) -> ()
      }
      event "Save to POSCAR": Value Change {
        n163 = event-data() -> ()  [unwired: 1 in, 5 out]
        n164 = call "File Dialog"() -> ("selected path"=w221:path)  [unwired: 12 in, 3 out]
        n165 = Build Path(base path=w221, name or relative path="Structure Name") -> (appended path=w219:path)
        n166 = Create Folder(path (use dialog)=w219) -> (created path=w218:path)  [unwired: 2 in, 2 out]
        n167 = stacked-sequence {
          tunnel: "Structure Name" -> [w223 _]
          tunnel: w218 -> [w222 w263]
          frame #0 {
            n168 = local read "Grain Boundary"() -> (w228:T1)
            n169 = Build Path(base path=w222, name or relative path="POSCAR") -> (appended path=w225:path)
            n170 = Bundle By Name(cluster=w228, "Structure Name"=w223) -> (w227:T1)
            n171 = call "Atoms to POSCAR.vi"("Atomic Structure"=w227) -> ("POSCAR File"=w224:string)  [unwired: 10 in]
            n172 = Write to Text File(file (use dialog)=w225, text=w224) -> ()  [unwired: 2 in, 3 out]
          }
          frame #1 {
            w238 = "," ("string")
            w235 = i16 2 ("precision (6)")
            w254 = "," ("string")
            w257 = "," ("string")
            n173 = local read "Grain 1 Orientation"() -> (w247:dbl[])
            n174 = local read "Grain 2 Orientation"() -> (w249:dbl[])
            n175 = local read "Translation Vector"() -> (w236:dbl[])
            n176 = Build Path(base path=w263, name or relative path="README.txt") -> (appended path=w265:path)
            n177 = Number To Fractional String(number=w247, precision (6)=w235) -> (F-format string=w246:string[])  [unwired: 2 in]
            n178 = Number To Fractional String(number=w249, precision (6)=w235) -> (F-format string=w248:string[])  [unwired: 2 in]
            n179 = Number To Fractional String(number=w236, precision (6)=w235) -> (F-format string=w241:string[])  [unwired: 2 in]
            n180 = local read "Overlap Region (A)"() -> (w233:dbl)
            n181 = local read "Add Tilt Angle"() -> (w251:dbl)
            n182 = Index Array(array=w246) -> (element #1=w259:string, element #2=w258:string, element #3=w256:string)  [unwired: 3 in]
            n183 = Index Array(array=w248) -> (element #1=w252:string, element #2=w253:string, element #3=w255:string)  [unwired: 3 in]
            n184 = Index Array(array=w241) -> (element #1=w240:string, element #2=w239:string, element #3=w237:string)  [unwired: 3 in]
            n185 = local read "Grain 1 Start"() -> (w231:dbl)
            n186 = local read "Twist Angle"() -> (w250:dbl)
            n187 = Concatenate Strings(w259, w257, w258, w257, w256) -> (w245:string)
            n188 = Concatenate Strings(w252, w254, w253, w254, w255) -> (w244:string)
            n189 = Number To Fractional String(number=w250) -> (F-format string=w243:string)  [unwired: 3 in]
            n190 = Number To Fractional String(number=w251) -> (F-format string=w242:string)  [unwired: 3 in]
            n191 = Concatenate Strings(w240, w238, w239, w238, w237) -> (w234:string)
            n192 = Number To Fractional String(number=w233) -> (F-format string=w232:string)  [unwired: 3 in]
            n193 = Number To Fractional String(number=w231) -> (F-format string=w230:string)  [unwired: 3 in]
            n194 = Build Array(w245, w244, w243, w242, w234, w232, w230) -> (w229:string[])
            n195 = Build Array(string[] ["Grain 1 Orientation", "Grain 2 Orientation", "Twist Angle (Degree)", "Tilt Angle (Degree)", "Translation (x,y,z)", "Overlap Length (A)", "Grain 1 Start (A)"], w229) -> (w261:string[][])
            n196 = Transpose 2D Array(2D array=w261) -> (transposed array=w260:string[][])
            n197 = call-poly <vilib>:"Write To Spreadsheet File.vi"("2D data"=w260, "file path (dialog if empty)"=w265) -> ()  [unwired: 6 in, 1 out]
          }
        }
      }
    }
  }
  n198 = call <vilib>:"Create Object.vi"("Name"="Base") -> ("Scene:New Object"=→"Grain 2 Object":refnum<vi>)  [unwired: 1 in, 9 out]
  n199 = call <vilib>:"Create Object.vi"("Name"="Base") -> ("Scene:New Object"=→"Grain 1 Object":refnum<vi>)  [unwired: 1 in, 9 out]
  n200 = call <vilib>:"Create Object.vi"("Name"="Base") -> ("Scene:New Object"=→"Grain Boundary Object":refnum<vi>)  [unwired: 1 in, 9 out]
  n201 = disable-structure shown="Disabled" {
    frame Disabled {
      n202 = local write "Conventional Unit Cell"(T1 {"Structure Name"="CdTe", "Lattice vector a"=[6.615785553057252, 0.0, 0.0], "Lattice vector b"=[0.0, 6.615785553057252, 0.0], "Lattice vector c"=[0.0, 0.0, 6.615785553057252], "Atoms Array"=[{"Atom Name"="Cd", "Positions (Direct)"=[[0.0, 0.0, 0.0], [0.0, 0.5, 0.5], [0.5, 0.0, 0.5], [0.5, 0.5, 0.0]], "Positions (Cartesian)"=[[0.0, 0.0, 0.0], [0.0, 3.307892776528626, 3.307892776528626], [3.307892776528626, 0.0, 3.307892776528626], [3.307892776528626, 3.307892776528626, 0.0]]}, {"Atom Name"="Te", "Positions (Direct)"=[[0.25, 0.25, 0.25], [0.75, 0.75, 0.25], [0.75, 0.25, 0.75], [0.25, 0.75, 0.75]], "Positions (Cartesian)"=[[1.653946388264313, 1.653946388264313, 1.653946388264313], [4.96183916479294, 4.96183916479294, 1.653946388264313], [4.96183916479294, 1.653946388264313, 4.96183916479294], [1.653946388264313, 4.96183916479294, 4.96183916479294]]}], "# of atoms"=8} ("Structure")) -> ()
    }
    frame Enabled {
    }
  }
